vi "L21.vi"() -> ()   [LabVIEW 2012]
panel:
  out "sum":i32
  out "Array":i32[](array[numeric])
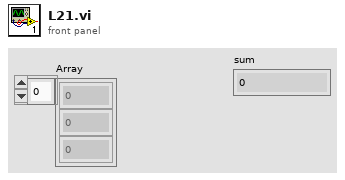
[diagram p1: front panel]
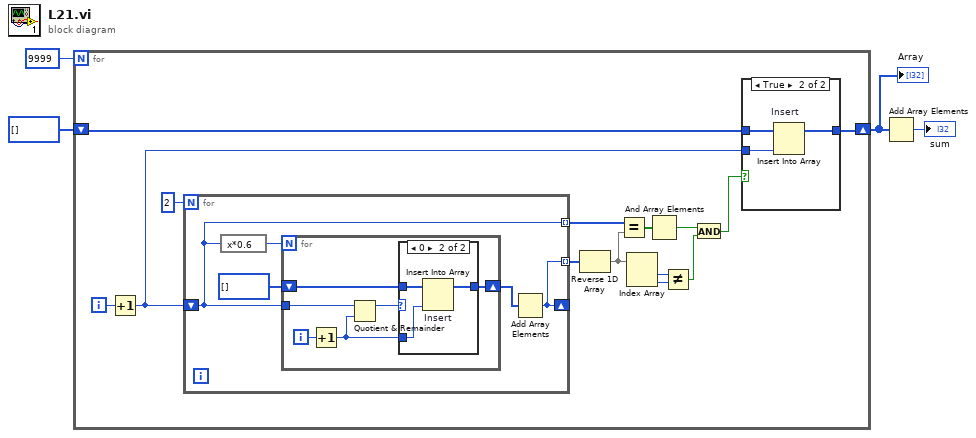
[diagram p0: block diagram]
diagram:
  n1 = for {
    N: 9999 -> [_]
    shift-right: [w13] -> w1
    shift-left: i32[] [] -> [w11]
    i -> [w14]
    n2 = Increment(x=w14) -> (x+1=w12:i32)
    n3 = for {
      N: 2 -> [_]
      shift-right: [w23] -> _
      shift-left: w12 -> [w24]
      tunnel: [w24] -> w16 mode=indexing
      tunnel: [w23] -> w17 mode=indexing
      n4 = expression code="x*0.6"(w24) -> (w27:i32)
      n5 = for {
        N: w27 -> [_]
        tunnel: w24 -> [w31]
        shift-right: [w29] -> w25
        shift-left: i32[] [] -> [w28]
        i -> [w33]
        n6 = Increment(x=w33) -> (x+1=w30:i32)
        n7 = Quotient & Remainder(x=w31, y=w30) -> (x-y*floor(x/y)=w32:i32)  [unwired: 1 out]
        n8 = case shown="0" w32 {
          tunnel: w30 -> [_ w37]
          tunnel: [w34 w36] -> w29
          tunnel: w28 -> [w34 w35]
          frame Default {
          }
          frame 0 {
            n9 = Insert Into Array "Insert"(array=w35, new element=w37) -> (w36:i32[])  [unwired: 1 in]
          }
        }
      }
      n10 = Add Array Elements(numeric array=w25) -> (sum=w23:i32)
    }
    n11 = Reverse 1D Array(array=w17) -> (reversed array=w8:i32[])
    n12 = Equal?(x=w16, y=w8) -> (x = y?=w15:bool[])
    n13 = Index Array(array=w8) -> (element #1=w9:i32, element #2=w10:i32)  [unwired: 2 in]
    n14 = And Array Elements(Boolean array=w15) -> (logical AND=w6:bool)
    n15 = Not Equal?(x=w9, y=w10) -> (x != y?=w7:bool)
    n16 = And(x=w6, y=w7) -> (x .and. y?=w5:bool)
    n17 = case shown="True" w5 {
      tunnel: [w19 w22] -> w13
      tunnel: w12 -> [_ w21]
      tunnel: w11 -> [w19 w20]
      frame False {
      }
      frame True {
        n18 = Insert Into Array "Insert"(array=w20, new element=w21) -> (w22:i32[])  [unwired: 1 in]
      }
    }
  }
  "Array" <- w1
  n19 = Add Array Elements(numeric array=w1) -> (sum=→"sum":i32)
